vi "Add Event.vi"(8 "error in (no error)":errorcluster, 9 "Insert At":i32, 10 "Name":string, 11 "Tosca in":refnum<class "Parameters.lvclass">) -> (0 "error out":errorcluster, 3 "Tosca out":refnum<class "Parameters.lvclass">)   [LabVIEW 2020, in "Parameters.lvclass"]
uses:
  Parameters.lvclass
  Parameters.lvclass/Parameters.ctl
  Digital Input VIs/Tosca-Input Event.ctl
  Digital Input VIs/Tosca-Input Criterion.ctl
  epl-vi-lib/Utility VIs/Type Defs/Logic State.ctl
  Typedefs/Tosca-Accumulator.ctl
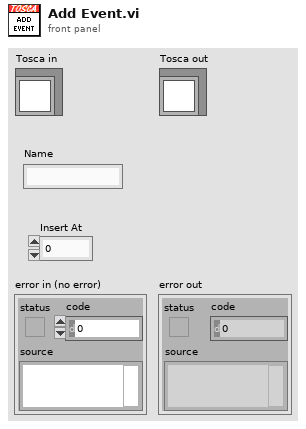
[diagram p1: front panel]
types:
  T1 = typedef "Tosca-Input Criterion.ctl" = cluster{"DigInput":i32, "State":T2, "Time (ms)":i32, "Name":string}
  T2 = typedef "Logic State.ctl" = enum16{"Low", "High", "Rising", "Falling"}
  T3 = typedef "Tosca-Input Event.ctl" = cluster{"Name":string, "Criteria":T1[], "Operators":enum16{"AND", "OR"}[], "Accumulator":T4}
  T4 = typedef "Tosca-Accumulator.ctl" = cluster{"active":bool, "N":i32, "T":dbl, "Imax":dbl, "latency":dbl}
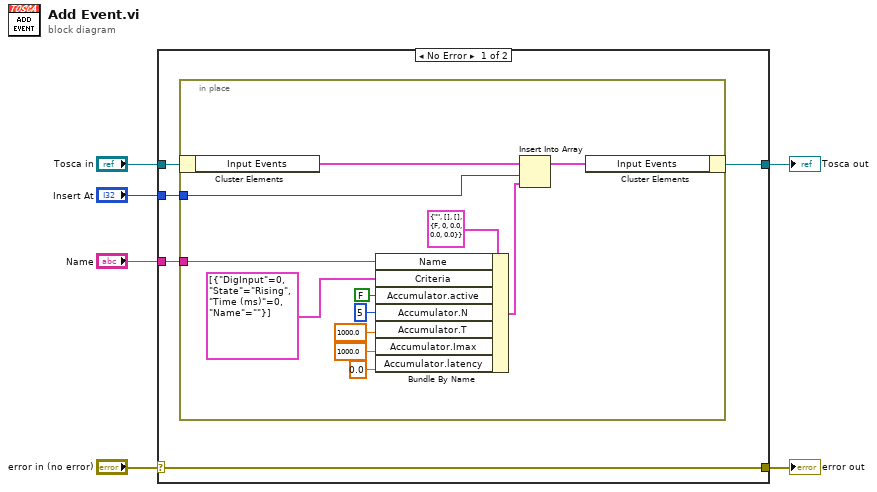
[diagram p0: block diagram]
diagram:
  n1 = case shown="No Error" "error in (no error)" {
    selector: "error in (no error)" -> [w11 w25]
    tunnel: [w11 w25] -> w5
    tunnel: [w9 w24] -> w3
    tunnel: "Tosca in" -> [w10 w24]
    tunnel: "Insert At" -> [w8 _]
    tunnel: "Name" -> [w7 _]
    frame No Error {
      n2 = in-place {
        in-place-border: w8 -> [w21]
        in-place-border: w7 -> [w18]
        n3 = in-place-cluster #1(w10) -> ("Input Events"=w23:T3[])
        n4 = Bundle By Name(cluster=T3 {"Name"="", "Criteria"=[], "Operators"=[], "Accumulator"={"active"=FALSE, "N"=0, "T"=0.0, "Imax"=0.0, "latency"=0.0}} ("new element/subarray"), "Name"=w18, "Criteria"=T1[] [{"DigInput"=0, "State"=enum."Rising", "Time (ms)"=0, "Name"=""}], "Accumulator.active"=FALSE, "Accumulator.N"=5, "Accumulator.T"=1000.0, "Accumulator.Imax"=1000.0, "Accumulator.latency"=0.0) -> (w19:T3)
        n5 = Insert Into Array(array=w23, index=w21, new element=w19) -> (w22:T3[])
        n6 = in-place-cluster #1("Input Events"=w22) -> (w9:refnum<class "Parameters.lvclass">)
      }
    }
    frame Error {
    }
  }
  "error out" <- w5
  "Tosca out" <- w3
